vi "custom_picktime.vi"(7 "first":i32=1, 8 "wdnames":string[](array[string])=["Sun", "Mon", "Tue", "Wed", "Thu", "Fri", "Sat"], 9 "fmtstr":string="%<%.3X\n%x>T", 10 "secin":timestamp, 11 "mnames":string[](array[string])=["January", "February", "March", "April", "May", "June", "July", "August", "September", "October", "November", "December"]) -> (1 "ok":bool, 2 "secout":timestamp format="%<%Z>T")   [LabVIEW 2019]
uses:
  AULocalize/SubVIs/RegisterVI.vi
  AULocalize/SubVIs/Get Localized Phrase Compact Interface 1D.vi
panel:
  in  "custom_time_display":timestamp format="%<%x %H:%M:%S>T"
  out "DaylightSavingState":string
  out "date time rec":T1
  in  "Time Display":timestamp format="%<%.3X>T"
  in  "now":bool
  in  "cancel":bool
  in  "ok":bool
  in  "Year":i32=1905 caption="(ий)Year" min=1600 max=3000
  in  "Month":i32(ring) caption="(ий)Month" items=["(ий)January", "(ий)February", "(ий)March", "(ий)April", "(ий)May", "(ий)June", "(ий)July", "(ий)August", "(ий)September", "(ий)October", "(ий)November", "(ий)December"]
  in  "Date":i32(listbox) caption="(ий)Date"
  # "(0 for Sunday, 1 for Monday, etc)"
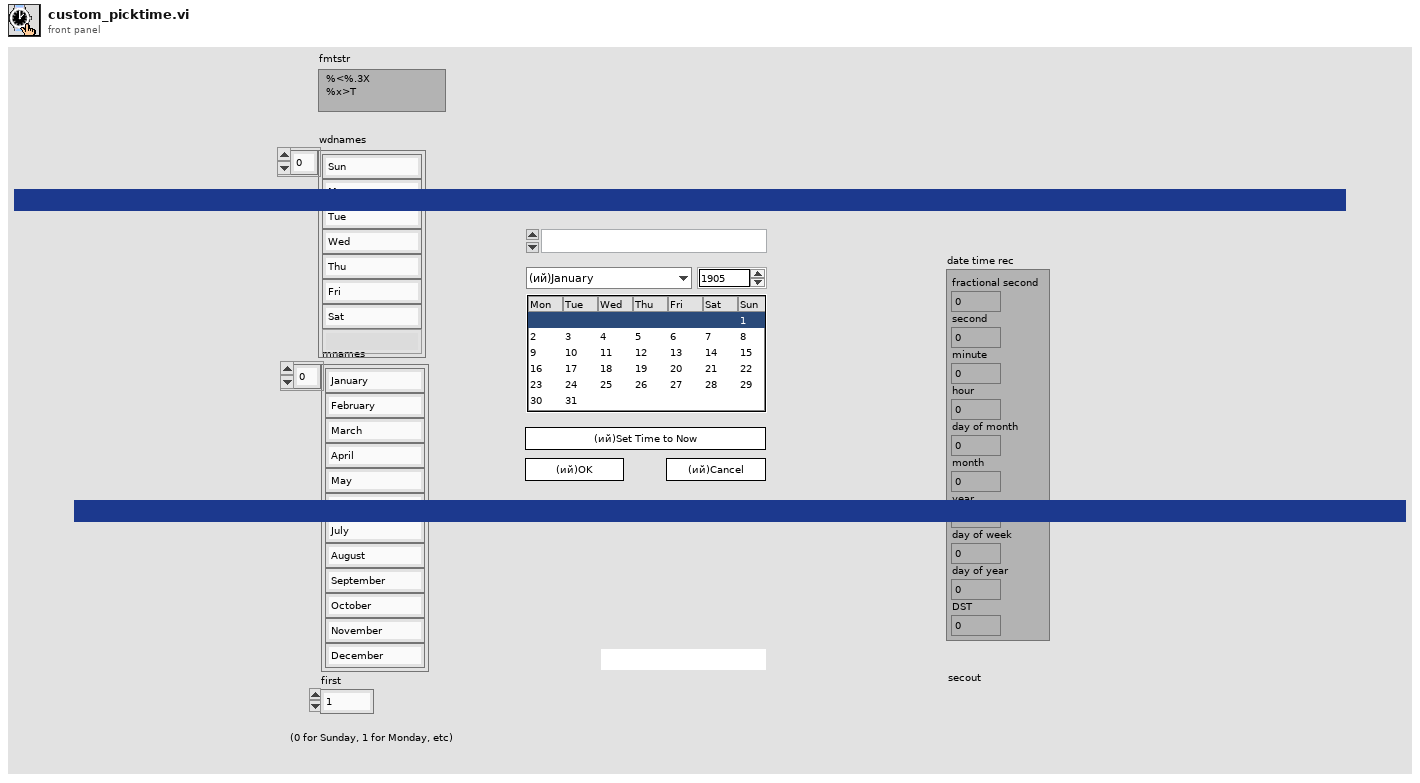
[diagram p1: front panel]
types:
  T1 = cluster{"fractional second":dbl, "second":i32, "minute":i32, "hour":i32, "day of month":i32, "month":i32, "year":i32, "day of week":i32, "day of year":i32, "DST":i32}
  T2 = typedef "LVDateTimeRec.ctl" = cluster{"fractional second":dbl, "second":i32, "minute":i32, "hour":i32, "day of month":i32, "month":i32, "year":i32, "day of week":i32, "day of year":i32, "DST":i32}
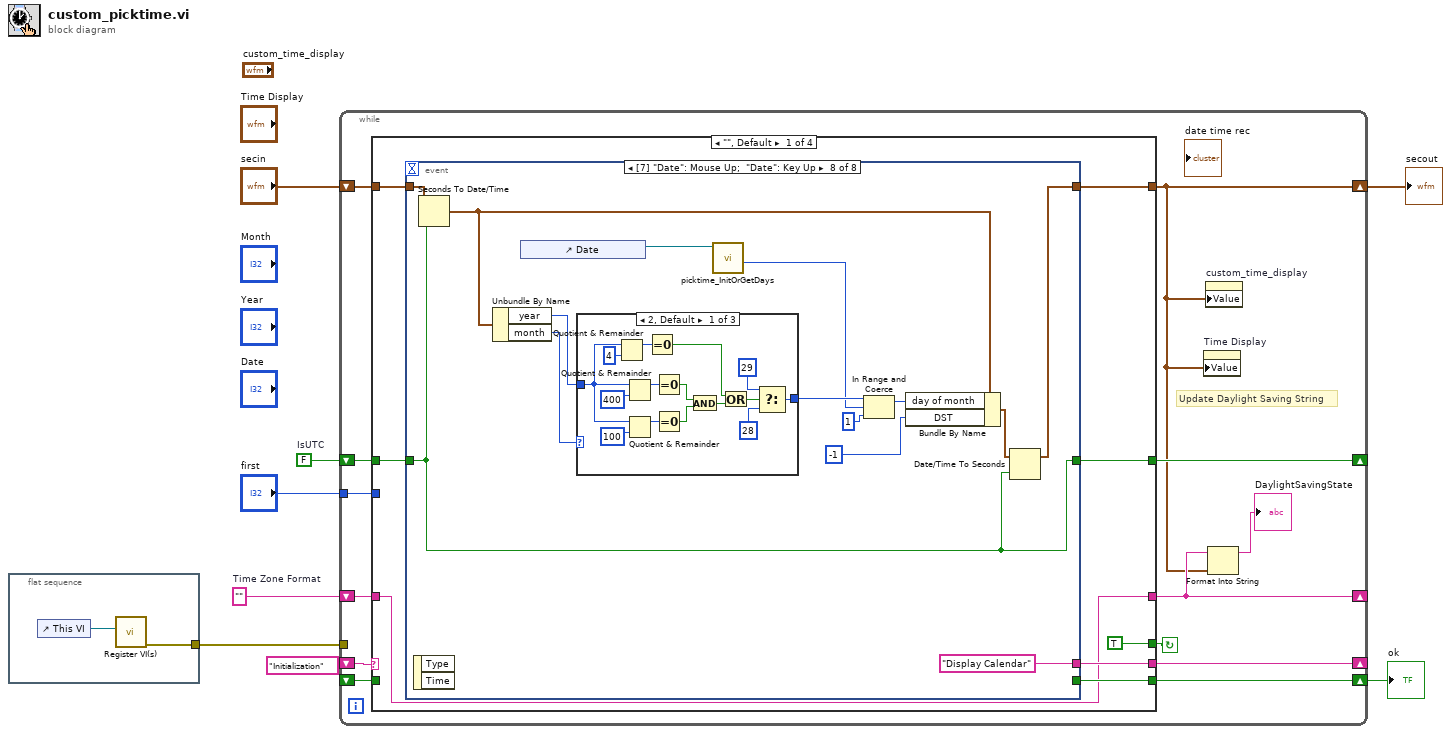
[diagram p0: block diagram]
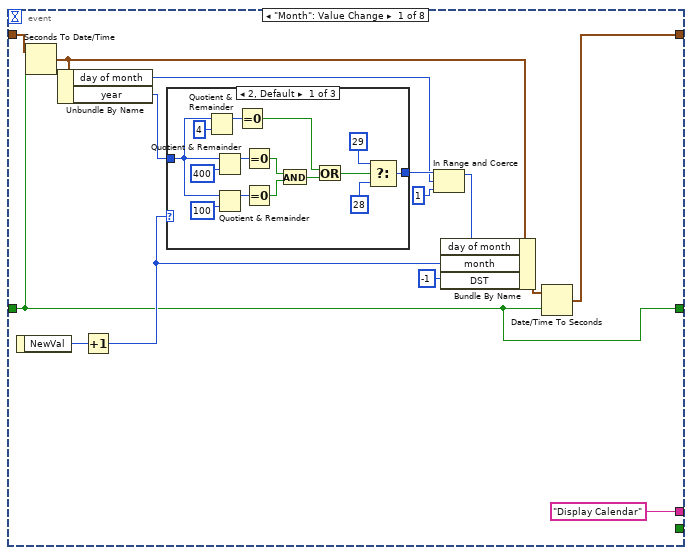
[diagram p2: hidden frame]
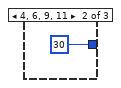
[diagram p3: hidden frame]
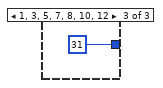
[diagram p4: hidden frame]
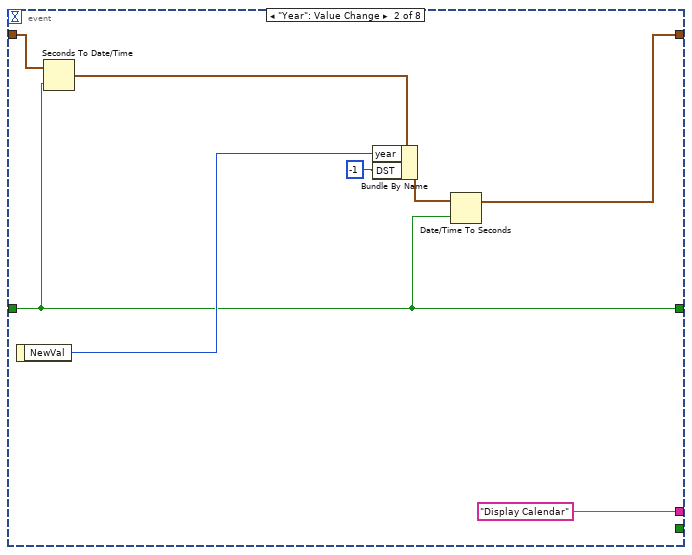
[diagram p5: hidden frame]
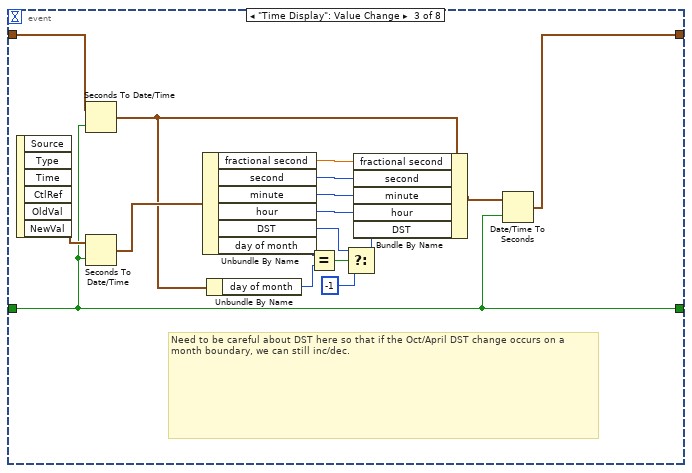
[diagram p6: hidden frame]
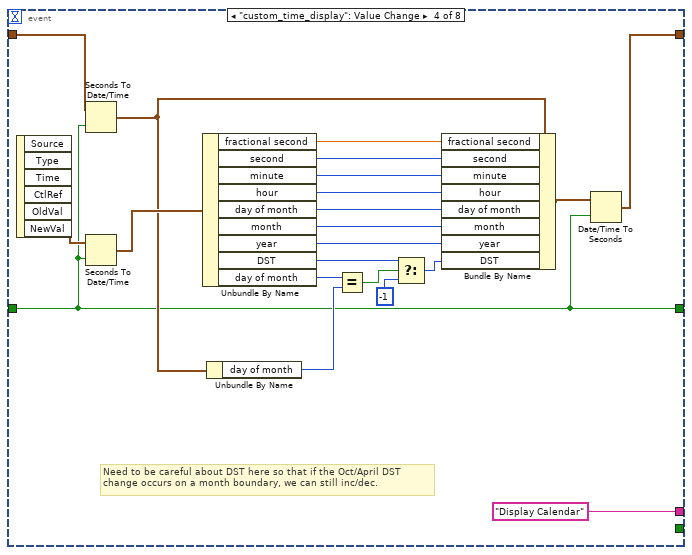
[diagram p7: hidden frame]
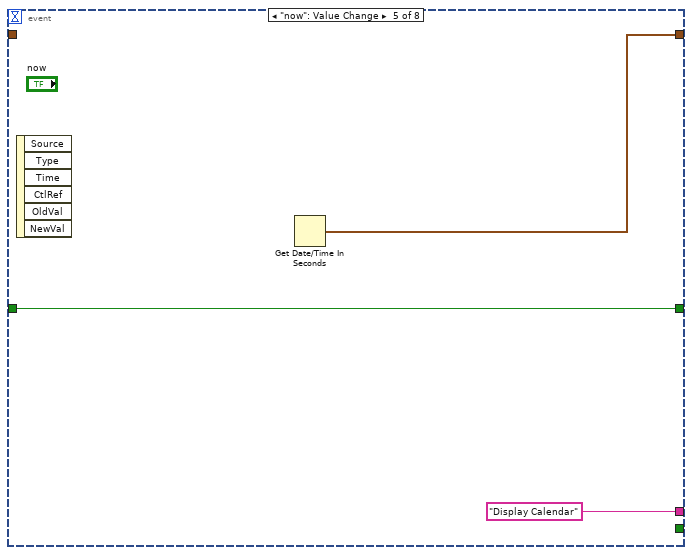
[diagram p8: hidden frame]
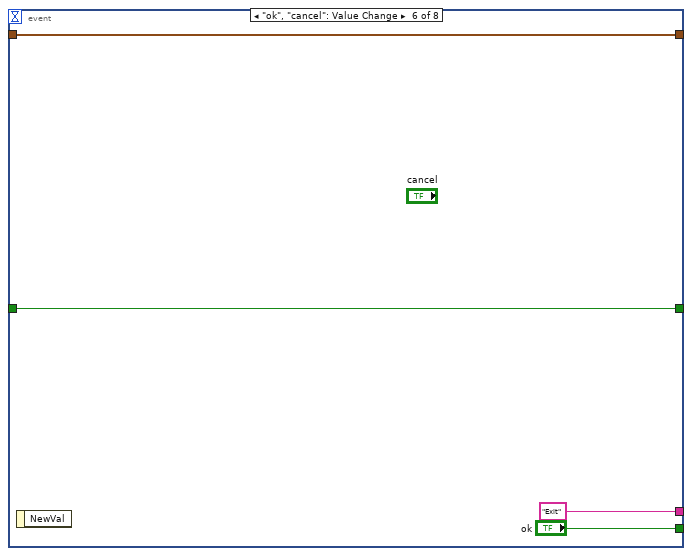
[diagram p9: hidden frame]
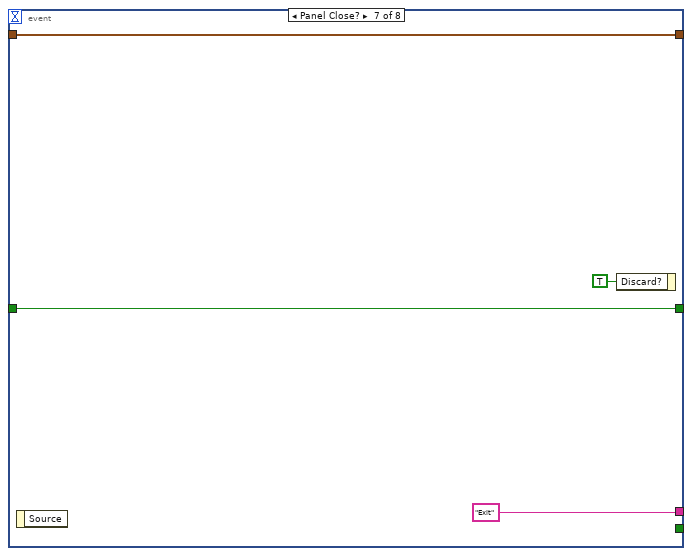
[diagram p10: hidden frame]
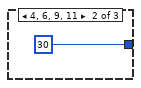
[diagram p11: hidden frame]
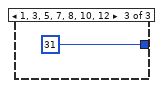
[diagram p12: hidden frame]
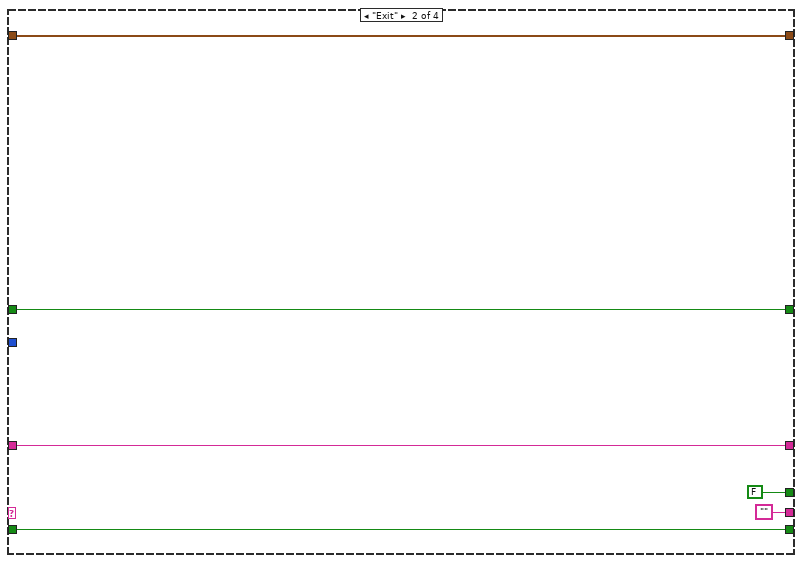
[diagram p13: hidden frame]
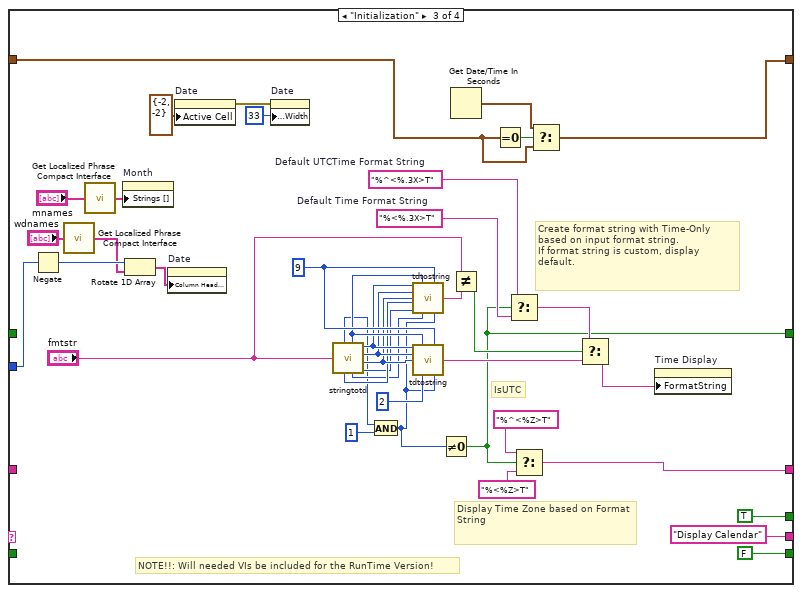
[diagram p14: hidden frame]
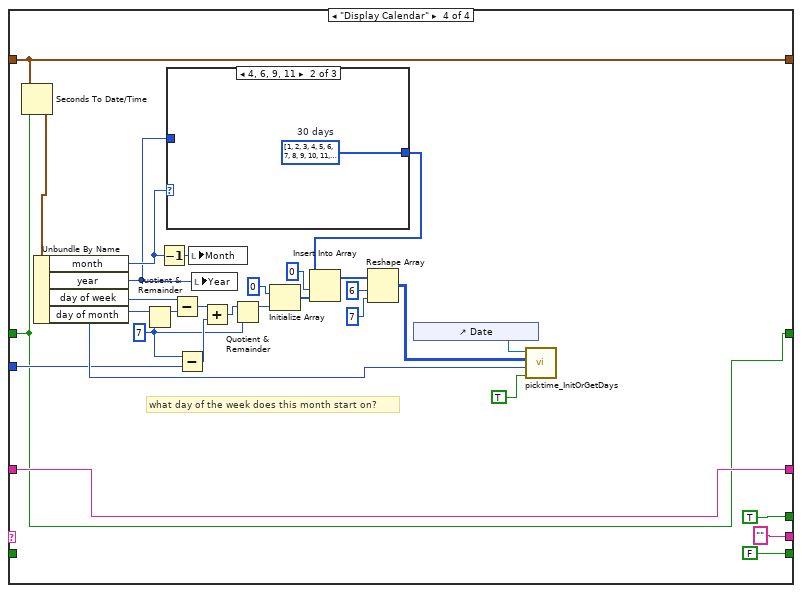
[diagram p15: hidden frame]
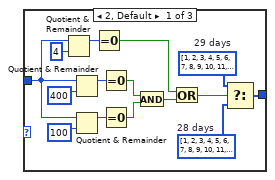
[diagram p16: hidden frame]
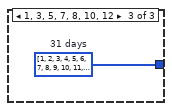
[diagram p17: hidden frame]
diagram:
  w3 = FALSE  # IsUTC
  w5 = ""  # Time Zone Format
  n1 = flat-sequence {
    tunnel: [w9] -> w1
    frame #0 {
      n2 = control-ref of="This VI"() -> (w10:refnum<vi>)
      n3 = call-poly "Register VI(s).vi"("VI Ref"=w10) -> ("error out"=w9:errorcluster)  [unwired: 9 in, 1 out]
    }
  }
  n4 = while {
    shift-right: [w22] -> _
    shift-left: "Initialization" -> [w23]
    shift-right: [w11] -> w2
    shift-left: "secin" -> [w21]
    shift-right: [w19] -> w7
    shift-left: _ -> [w18]
    shift-right: [w15] -> _
    shift-left: w5 -> [w17]
    tunnel: "first" -> [w14]
    shift-right: [w12] -> _
    shift-left: w3 -> [w13]
    tunnel: w1 -> [_]
    stop <- w20 continue-if-true
    # "Update Daylight Saving String"
    n5 = case shown="\"\", Default" w23 {
      tunnel: [w28 "" "Display Calendar" ""] -> w22
      tunnel: [TRUE FALSE TRUE TRUE] -> w20
      tunnel: w21 -> [w29 w153 w188 w208]
      tunnel: [w30 w153 w187 w208] -> w11
      tunnel: [w27 w154 FALSE ("ok") FALSE ("ok")] -> w19
      tunnel: w18 -> [_ w154 _ _]
      tunnel: [w26 w152 w167 w207] -> w15
      tunnel: w17 -> [w26 w152 _ w207]
      tunnel: w14 -> [_ _ w163 w203]
      tunnel: w13 -> [w25 w151 _ w200]
      tunnel: [w24 w151 w161 w200] -> w12
      frame "", Default {
        n6 = event shown="[7] \"Date\": Mouse Up;  \"Date\": Key Up" {
          selector: _ -> [_ _ _ _ _ _ _ _]
          dyn-events: _ -> [_ _ _ _ _ _ _ _]
          timeout: _ -> [_ _ _ _ _ _ _ _]
          tunnel: w29 -> [w35 w66 w86 w107 _ w113 w118 w125]
          tunnel: [w34 w64 w84 w105 w110 w113 w118 w123] -> w30
          tunnel: ["Display Calendar" "Display Calendar" _ "Display Calendar" "Display Calendar" "Exit" "Exit" "Display Calendar"] -> w28
          tunnel: [_ _ _ _ _ "ok" _ _] -> w27
          tunnel: w25 -> [w32 w63 w71 w92 w109 w112 w117 w122]
          tunnel: [w32 w63 w71 w92 w109 w112 w117 w122] -> w24
          event "Month": Value Change {
            n7 = event-data() -> ("NewVal"=w45:i32)  [unwired: 1 out]
            n8 = Seconds To Date/Time(time stamp (now)=w35, to UTC (F)=w32) -> (date time rec=w33:T2)
            n9 = Unbundle By Name(w33) -> ("day of month"=w39:i32, "year"=w40:i32)
            n10 = Increment(x=w45) -> (x+1=w43:i32)
            n11 = case shown="2, Default" w43 {
              tunnel: [w58 30 31] -> w42
              tunnel: w40 -> [w53 _ _]
              frame 2, Default {
                n12 = Quotient & Remainder(x=w53, y=4) -> (x-y*floor(x/y)=w57:i32)  [unwired: 1 out]
                n13 = Quotient & Remainder(x=w53, y=400) -> (x-y*floor(x/y)=w52:i32)  [unwired: 1 out]
                n14 = Quotient & Remainder(x=w53, y=100) -> (x-y*floor(x/y)=w51:i32)  [unwired: 1 out]
                n15 = Equal To 0?(x=w57) -> (x = 0?=w56:bool)
                n16 = Equal To 0?(x=w52) -> (x = 0?=w49:bool)
                n17 = Equal To 0?(x=w51) -> (x = 0?=w50:bool)
                n18 = And(x=w49, y=w50) -> (x .and. y?=w48:bool)
                n19 = Or(x=w56, y=w48) -> (x .or. y?=w55:bool)
                n20 = Select(t=29, s=w55, f=28) -> (s? t:f=w58:i32)
              }
              frame 4, 6, 9, 11 {
              }
              frame 1, 3, 5, 7, 8, 10, 12 {
              }
            }
            n21 = In Range and Coerce(upper limit=w42, x=w39, lower limit=1) -> (coerced(x)=w38:i32)  [unwired: 1 out]
            n22 = Bundle By Name(cluster=w33, "day of month"=w38, "month"=w43, "DST"=-1) -> (w37:T2)
            n23 = Date/Time To Seconds(1:w32, 2:w37) -> (0:w34:timestamp)
          }
          event "Year": Value Change {
            n24 = event-data() -> ("NewVal"=w70:i32)  [unwired: 1 out]
            n25 = Seconds To Date/Time(time stamp (now)=w66, to UTC (F)=w63) -> (date time rec=w65:T2)
            n26 = Bundle By Name(cluster=w65, "year"=w70, "DST"=-1) -> (w68:T2)
            n27 = Date/Time To Seconds(1:w63, 2:w68) -> (0:w64:timestamp)
          }
          event "Time Display": Value Change {
            # "Need to be careful about DST here so that if the Oct/April DST change occurs on a month boundary, we can still inc/dec."
            n28 = event-data() -> ("NewVal"=w87:timestamp)  [unwired: 6 out]
            n29 = Seconds To Date/Time(time stamp (now)=w86, to UTC (F)=w71) -> (date time rec=w74:T2)
            n30 = Seconds To Date/Time(time stamp (now)=w87, to UTC (F)=w71) -> (date time rec=w83:T2)
            n31 = Unbundle By Name(w83) -> ("fractional second"=w79:dbl, "second"=w80:i32, "minute"=w81:i32, "hour"=w82:i32, "DST"=w76:i32, "day of month"=w72:i32)
            n32 = Unbundle By Name(w74) -> ("day of month"=w73:i32)
            n33 = Equal?(x=w72, y=w73) -> (x = y?=w78:bool)
            n34 = Select(t=w76, s=w78, f=-1) -> (s? t:f=w75:i32)
            n35 = Bundle By Name(cluster=w74, "fractional second"=w79, "second"=w80, "minute"=w81, "hour"=w82, "DST"=w75) -> (w85:T2)
            n36 = Date/Time To Seconds(1:w71, 2:w85) -> (0:w84:timestamp)
          }
          event "custom_time_display": Value Change {
            # "Need to be careful about DST here so that if the Oct/April DST change occurs on a month boundary, we can still inc/dec."
            n37 = event-data() -> ("NewVal"=w108:timestamp)  [unwired: 6 out]
            n38 = Seconds To Date/Time(time stamp (now)=w107, to UTC (F)=w92) -> (date time rec=w95:T2)
            n39 = Seconds To Date/Time(time stamp (now)=w108, to UTC (F)=w92) -> (date time rec=w104:T2)
            n40 = Unbundle By Name(w104) -> ("fractional second"=w100:dbl, "second"=w101:i32, "minute"=w102:i32, "hour"=w103:i32, "day of month"=w90:i32, "month"=w89:i32, "year"=w88:i32, "DST"=w97:i32, "day of month"=w93:i32)
            n41 = Unbundle By Name(w95) -> ("day of month"=w94:i32)
            n42 = Equal?(x=w93, y=w94) -> (x = y?=w99:bool)
            n43 = Select(t=w97, s=w99, f=-1) -> (s? t:f=w96:i32)
            n44 = Bundle By Name(cluster=w95, "fractional second"=w100, "second"=w101, "minute"=w102, "hour"=w103, "day of month"=w90, "month"=w89, "year"=w88, "DST"=w96) -> (w106:T2)
            n45 = Date/Time To Seconds(1:w92, 2:w106) -> (0:w105:timestamp)
          }
          event "now": Value Change {
            n46 = event-data() -> ()  [unwired: 7 out]
            n47 = Get Date/Time In Seconds() -> (seconds since 1Jan1904=w110:timestamp)
          }
          event "ok", "cancel": Value Change {
            n48 = event-data() -> ()  [unwired: 2 out]
          }
          event Panel Close? {
            n49 = event-data() -> ()  [unwired: 2 out]
            n50 = event-data("Discard?"=TRUE) -> ()  [unwired: 1 in, 1 out]
          }
          event "Date": Mouse Up; "Date": Key Up {
            n51 = event-data() -> ()  [unwired: 3 out]
            n52 = Seconds To Date/Time(time stamp (now)=w125, to UTC (F)=w122) -> (date time rec=w124:T2)
            n53 = Unbundle By Name(w124) -> ("year"=w131:i32, "month"=w130:i32)
            n54 = control-ref of="Date"() -> (w120:refnum<vi>)
            n55 = case shown="2, Default" w130 {
              tunnel: [w146 30 31] -> w133
              tunnel: w131 -> [w141 _ _]
              frame 2, Default {
                n56 = Quotient & Remainder(x=w141, y=4) -> (x-y*floor(x/y)=w145:i32)  [unwired: 1 out]
                n57 = Quotient & Remainder(x=w141, y=400) -> (x-y*floor(x/y)=w140:i32)  [unwired: 1 out]
                n58 = Quotient & Remainder(x=w141, y=100) -> (x-y*floor(x/y)=w139:i32)  [unwired: 1 out]
                n59 = Equal To 0?(x=w145) -> (x = 0?=w144:bool)
                n60 = Equal To 0?(x=w140) -> (x = 0?=w137:bool)
                n61 = Equal To 0?(x=w139) -> (x = 0?=w138:bool)
                n62 = And(x=w137, y=w138) -> (x .and. y?=w136:bool)
                n63 = Or(x=w144, y=w136) -> (x .or. y?=w143:bool)
                n64 = Select(t=29, s=w143, f=28) -> (s? t:f=w146:i32)
              }
              frame 4, 6, 9, 11 {
              }
              frame 1, 3, 5, 7, 8, 10, 12 {
              }
            }
            n65 = call <resource>:"picktime_InitOrGetDays.vi"("reference"=w120) -> ("day of month(out)"=w121:i32)  [unwired: 3 in, 7 out]
            n66 = In Range and Coerce(upper limit=w133, x=w121, lower limit=1) -> (coerced(x)=w129:i32)  [unwired: 1 out]
            n67 = Bundle By Name(cluster=w124, "day of month"=w129, "DST"=-1) -> (w127:T2)
            n68 = Date/Time To Seconds(1:w122, 2:w127) -> (0:w123:timestamp)
          }
        }
      }
      frame "Exit" {
      }
      frame "Initialization" {
        w170 = "%^<%.3X>T"  # Default UTCTime Format String
        w169 = "%<%.3X>T"  # Default Time Format String
        w183 = 9 ("Type (9 = Absolute)")
        # "IsUTC"
        # "Display Time Zone based on Format String"
        # "NOTE!!: Will needed VIs be included for the RunTime Version!"
        # "Create format string with Time-Only based on input format string.\nIf format string is custom, display default."
        n69 = Negate(x=w163) -> (-x=w162:i32)
        n70 = call-poly "Get Localized Phrase Compact Interface.vi"("Key"="wdnames") -> ("Translated Phrase"=w157:string[])
        n71 = call-poly "Get Localized Phrase Compact Interface.vi"("Key"="mnames") -> ("Translated Phrase"=w158:string[])
        n72 = property on="Month" class="Ring (strict)"("Strings []"=w158) -> ()  [unwired: 2 in, 2 out]
        n73 = Rotate 1D Array(1:w157, 2:w162) -> (0:w165:string[])
        n74 = property on="Date" class="MCListbox (strict)"("Column Header Strings[]"=w165) -> ()  [unwired: 2 in, 2 out]
        n75 = property on="Date" class="MCListbox (strict)"("Active Cell"=cluster{i32, i32} {-2, -2}) -> (error out=w195:errorcluster)  [unwired: 2 in, 1 out]
        n76 = property on="Date" class="MCListbox (strict)"(error in=w195, "Cell Size:Width"=u32 33) -> ()  [unwired: 1 in, 2 out]
        n77 = call <resource>:"stringtotd.vi"("Time & Date Format String"="fmtstr") -> ("UTC"=w159:i16, "MDY"=w178:i16, "Time Format"=w182:i16, "AM/PM"=w181:i16, "included seconds"=w180:i16, "Date Format"=w176:i16, "seconds precision"=w179:i16, "Year Format"=w177:i16)  [unwired: 2 out]
        n78 = And(x=w159, y=i16 1) -> (x .and. y?=w160:i16)
        n79 = call <resource>:"tdtostring.vi"("AM/PM"=w181, "Time Format"=w182, "Type (10 = Absolute)"=w183, "included seconds"=w180, "seconds precision"=w179, "m-d-y sequence"=w178, "year format"=w177, "Date Format"=w176, "UTC"=w160) -> ("Format String"=w174:string)  [unwired: 2 in, 4 out]
        n80 = call <resource>:"tdtostring.vi"("AM/PM"=w181, "Time Format"=w182, "Type (10 = Absolute)"=w183, "included seconds"=w180, "seconds precision"=w179, "Date Format"=i16 2, "UTC"=w160) -> ("Format String"=w172:string)  [unwired: 4 in, 4 out]
        n81 = Not Equal To 0?(x=w160) -> (x != 0?=w161:bool)
        n82 = Get Date/Time In Seconds() -> (seconds since 1Jan1904=w190:timestamp)
        n83 = Not Equal?(x="fmtstr", y=w174) -> (x != y?=w173:bool)
        n84 = Equal To 0?(x=w188) -> (x = 0?=w191:bool)
        n85 = Select(t=w170, s=w161, f=w169) -> (s? t:f=w168:string)
        n86 = Select(t="%^<%Z>T", s=w161, f="%<%Z>T") -> (s? t:f=w167:string)
        n87 = Select(t=w190, s=w191, f=w188) -> (s? t:f=w187:timestamp)
        n88 = Select(t=w168, s=w173, f=w172) -> (s? t:f=w171:string)
        n89 = property on="Time Display" class="AbsTime (strict)"("FormatString"=w171) -> ()  [unwired: 2 in, 2 out]
      }
      frame "Display Calendar" {
        w201 = 7 ("y")
        # "what day of the week does this month start on?"
        n90 = Seconds To Date/Time(time stamp (now)=w208, to UTC (F)=w200) -> (date time rec=w209:T2)
        n91 = Unbundle By Name(w209) -> ("month"=w215:i32, "year"=w214:i32, "day of week"=w225:i32, "day of month"=w206:i32)
        n92 = Quotient & Remainder(x=w206, y=w201) -> (x-y*floor(x/y)=w224:i32)  [unwired: 1 out]
        n93 = Decrement(x=w215) -> (x-1=w216:i32)
        n94 = case shown="4, 6, 9, 11" w215 {
          tunnel: [w239 w242 w243] -> w210
          tunnel: w214 -> [w232 _ _]
          frame 2, Default {
            w237 = i32[] [1, 2, 3, 4, 5, 6, 7, 8, 9, 10, 11, 12, 13, 14, 15, 16, 17, 18, 19, 20, 21, 22, 23, 24, 25, 26, 27, 28]  # 28 days
            w238 = i32[] [1, 2, 3, 4, 5, 6, 7, 8, 9, 10, 11, 12, 13, 14, 15, 16, 17, 18, 19, 20, 21, 22, 23, 24, 25, 26, 27, 28, 29]  # 29 days
            n95 = Quotient & Remainder(x=w232, y=4) -> (x-y*floor(x/y)=w236:i32)  [unwired: 1 out]
            n96 = Quotient & Remainder(x=w232, y=400) -> (x-y*floor(x/y)=w231:i32)  [unwired: 1 out]
            n97 = Quotient & Remainder(x=w232, y=100) -> (x-y*floor(x/y)=w230:i32)  [unwired: 1 out]
            n98 = Equal To 0?(x=w236) -> (x = 0?=w235:bool)
            n99 = Equal To 0?(x=w231) -> (x = 0?=w228:bool)
            n100 = Equal To 0?(x=w230) -> (x = 0?=w229:bool)
            n101 = And(x=w228, y=w229) -> (x .and. y?=w227:bool)
            n102 = Or(x=w235, y=w227) -> (x .or. y?=w234:bool)
            n103 = Select(t=w238, s=w234, f=w237) -> (s? t:f=w239:i32[])
          }
          frame 4, 6, 9, 11 {
            w242 = i32[] [1, 2, 3, 4, 5, 6, 7, 8, 9, 10, 11, 12, 13, 14, 15, 16, 17, 18, 19, 20, 21, 22, 23, 24, 25, 26, 27, 28, 29, 30]  # 30 days
          }
          frame 1, 3, 5, 7, 8, 10, 12 {
            w243 = i32[] [1, 2, 3, 4, 5, 6, 7, 8, 9, 10, 11, 12, 13, 14, 15, 16, 17, 18, 19, 20, 21, 22, 23, 24, 25, 26, 27, 28, 29, 30, 31]  # 31 days
          }
        }
        n104 = Subtract(x=w225, y=w224) -> (x-y=w205:i32)
        n105 = Subtract(x=w201, y=w203) -> (x-y=w202:i32)
        n106 = local write "Month"(w216) -> ()
        n107 = local write "Year"(w214) -> ()
        n108 = Add(x=w205, y=w202) -> (x+y=w204:i32)
        n109 = Quotient & Remainder(x=w204, y=w201) -> (x-y*floor(x/y)=w213:i32)  [unwired: 1 out]
        n110 = Initialize Array(0, w213) -> (w221:i32[])
        n111 = Insert Into Array(array=w210, index=0, new element=w221) -> (w219:i32[])
        n112 = Reshape Array(w219, 6 ("dimension size"), 7 ("dimension size")) -> (w212:i32[][])
        n113 = control-ref of="Date"() -> (w199:refnum<vi>)
        n114 = call <resource>:"picktime_InitOrGetDays.vi"("Init"=TRUE, "day of month"=w206, "31 days"=w212, "reference"=w199) -> ()  [unwired: 8 out]
      }
    }
    n115 = property on="Time Display" class="AbsTime (strict)"("Value"=w11) -> ()  [unwired: 2 in, 2 out]
    n116 = property on="custom_time_display" class="AbsTime (strict)"("Value"=w11) -> ()  [unwired: 2 in, 2 out]
    n117 = Format Into String(format string=w15, w11) -> (resulting string=→"DaylightSavingState":string)  [unwired: 2 in, 1 out]
  }
  "ok" <- w7
  "secout" <- w2
